vi "UTEZ.vi"() -> ()   [LabVIEW 2020]
uses:
  <vilib>/httpClient/LabVIEWHTTPClient.lvlib
panel:
  in  "?":bool
  out "Temperatura":dbl
  out "Humedad":dbl
  out "Humedad":dbl(knob) scale=0.0..100.0
  out "Teemperatura":dbl(slide) scale=0.0..100.0
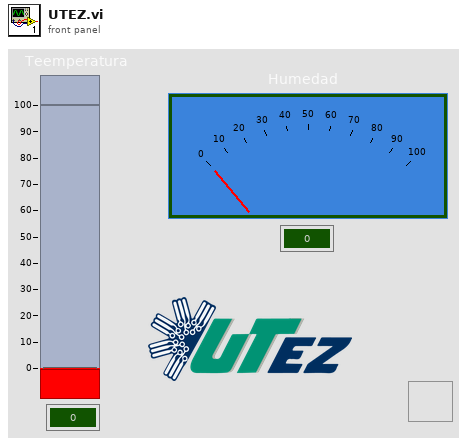
[diagram p1: front panel]
types:
  T1 = typedef "LabVIEWHTTPClient.lvlib/ClientHandle.ctl" = refnum<k1>
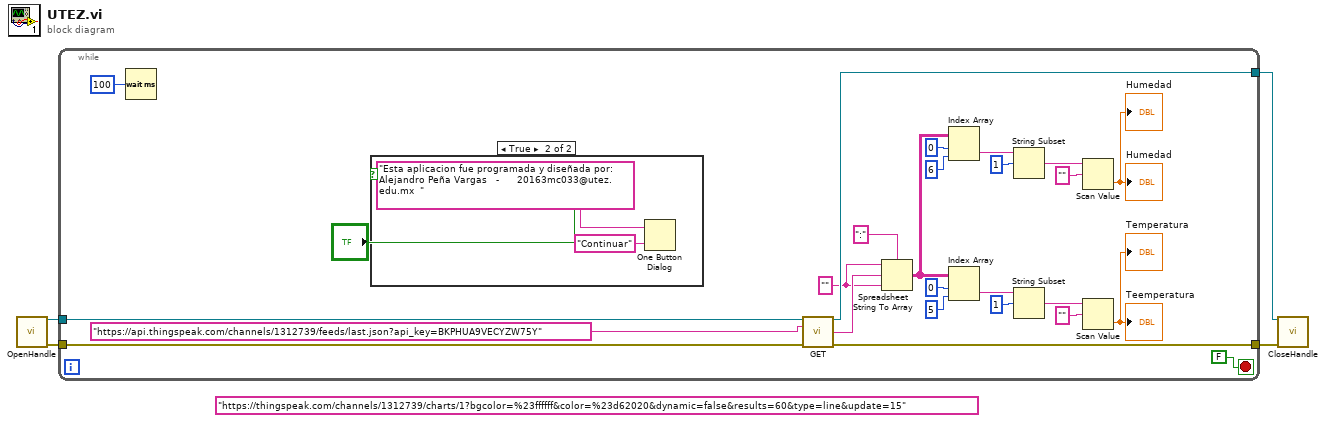
[diagram p0: block diagram]
diagram:
  (unwired) "https://thingspeak.com/channels/1312739/charts/1?bgcolor=%23ffffff&color=%23d62020&dynamic=false&results=60&type=line&update=15" ("URL")
  n1 = call <vilib>:"OpenHandle.vi"() -> ("client handle out"=w4:T1, "error out"=w2:errorcluster)  [unwired: 14 in]
  n2 = while {
    tunnel: w4 -> [w28]
    tunnel: [w27] -> w3
    tunnel: w2 -> [w26]
    tunnel: [w25] -> w1
    stop <- FALSE stop-if-true
    w21 = "" ("format string")
    n3 = Wait (ms)(milliseconds to wait=u32 100) -> ()  [unwired: 1 out]
    n4 = case shown="True" "?" {
      frame False {
      }
      frame True {
        n5 = One Button Dialog(message="Esta aplicacion fue programada y diseñada por: Alejandro Peña Vargas   -      20163mc033@utez.edu.mx  ", button name ("OK")="Continuar") -> ()  [unwired: 1 out]
      }
    }
    n6 = call <vilib>:"GET.vi"("client handle"=w28, "url"="https://api.thingspeak.com/channels/1312739/feeds/last.json?api_key=BKPHUA9VECYZW75Y" ("unescaped string in"), "error in (no error)"=w26) -> ("client handle out"=w27:T1, "body"=w22:string, "error out"=w25:errorcluster)  [unwired: 9 in, 1 out]
    n7 = Spreadsheet String To Array(delimiter (Tab)=":", format string=w21, spreadsheet string=w22, array type (2D Dbl)=w21) -> (array=w8:string[][])
    n8 = Index Array(array=w8, index (row)=0 ("disabled index (row)"), index (col)=6 ("disabled index (col)")) -> (element=w18:string)
    n9 = Index Array(array=w8, index (row)=0 ("disabled index (row)"), index (col)=5 ("disabled index (col)")) -> (element=w11:string)
    n10 = String Subset(string=w18, offset (0)=1) -> (substring=w16:string)  [unwired: 1 in]
    n11 = String Subset(string=w11, offset (0)=1) -> (substring=w13:string)  [unwired: 1 in]
    n12 = Scan Value(string=w16, format string="") -> (value=→"Humedad" →"Humedad":dbl)  [unwired: 1 in, 1 out]
    n13 = Scan Value(string=w13, format string="") -> (value=→"Teemperatura" →"Temperatura":dbl)  [unwired: 1 in, 1 out]
  }
  n14 = call <vilib>:"CloseHandle.vi"("client handle"=w3, "error in (no error)"=w1) -> ()  [unwired: 13 in, 1 out]
